vi "Get Enum Size.vi"(4 "Enum":variant) -> (1 "Size":i32)   [LabVIEW 2018, in "Potentiostat Galvanostat.lvclass"]
uses:
  Potentiostat Galvanostat.lvclass
  <vilib>/Utility/Data Type/NI_Data Type.lvlib
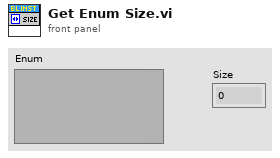
[diagram p1: front panel]
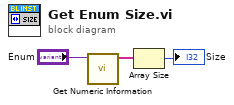
[diagram p0: block diagram]
diagram:
  n1 = call <vilib>:"Get Numeric Information.vi"("Variant"="Enum") -> ("Enum Names"=w1:string[])  [unwired: 7 in, 3 out]
  n2 = Array Size(array=w1) -> (size(s)=→"Size":i32)
